vi "Get Error Counter Channels.vi"(8 "error in":errorcluster, 11 "status section in":T1 format="%.0x") -> (0 "error out":errorcluster, 2 "error counter channel refs":T2={"general protocol"=18446744073709551615, "improper number of words"=18446744073709551615, "Manchester"=18446744073709551615, "monitor"=18446744073709551615, "parity"=18446744073709551615, "unconfigured frames"=18446744073709551615, "word"=18446744073709551615, "wrong sync"=18446744073709551615} {"wrong sync" format="%.0x"; "word" format="%.0x"; "unconfigured frames" format="%.0x"; "parity" format="%.0x"; "monitor" format="%.0x"; "Manchester" format="%.0x"; "improper number of words" format="%.0x"; "general protocol" format="%.0x"}, 3 "status section out":T1 format="%.0x")   [LabVIEW 2020, in "Ballard MIL-STD-1553 Scripting.lvlib"]
uses:
  <vilib>/NI VeriStand/Custom Device API/Custom Device Item Ref.ctl
  Constants.vi
  Ballard MIL-STD-1553 Scripting.lvlib
  <vilib>/NI VeriStand/Custom Device Tools/Custom Device Utility Library/Custom Device Utility Library.lvlib
  <vilib>/NI VeriStand/Custom Device Tools/Custom Device Utility Library/NI VeriStand - Search for Item by Name.vi
  <vilib>/NI VeriStand/Custom Device API/Custom Device API.lvlib
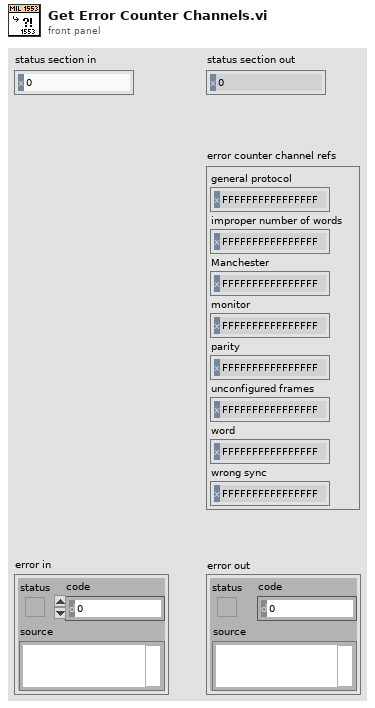
[diagram p1: front panel]
types:
  T1 = typedef "Custom Device API.lvlib/Custom Device Item Ref.ctl" = u64
  T2 = cluster{"general protocol":T1, "improper number of words":T1, "Manchester":T1, "monitor":T1, "parity":T1, "unconfigured frames":T1, "word":T1, "wrong sync":T1}
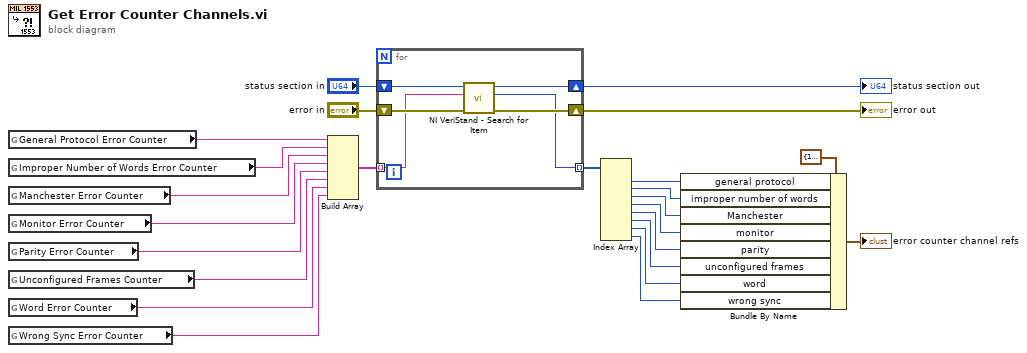
[diagram p0: block diagram]
diagram:
  n1 = global read "Constants.vi" "General Protocol Error Counter"() -> (w18:string)
  n2 = global read "Constants.vi" "Improper Number of Words Error Counter"() -> (w17:string)
  n3 = global read "Constants.vi" "Manchester Error Counter"() -> (w16:string)
  n4 = global read "Constants.vi" "Monitor Error Counter"() -> (w15:string)
  n5 = global read "Constants.vi" "Parity Error Counter"() -> (w14:string)
  n6 = global read "Constants.vi" "Unconfigured Frames Counter"() -> (w13:string)
  n7 = global read "Constants.vi" "Word Error Counter"() -> (w12:string)
  n8 = global read "Constants.vi" "Wrong Sync Error Counter"() -> (w11:string)
  n9 = Build Array(w18, w17, w16, w15, w14, w13, w12, w11) -> (w24:string[])
  n10 = for {
    shift-right: [w27] -> w20
    shift-left: "status section in" -> [w30]
    shift-right: [w28] -> w19
    shift-left: "error in" -> [w29]
    tunnel: w24 -> [w26] mode=indexing
    tunnel: [w25] -> w23 mode=indexing
    n11 = call-poly <vilib>:"NI VeriStand - Search for Item.vi"("error in"=w29, "Item Name"=w26, "Section Ref in"=w30) -> ("error out"=w28:errorcluster, "Item Ref"=w25:T1, "Section Ref out"=w27:T1)  [unwired: 5 in, 1 out]
  }
  "error out" <- w19
  "status section out" <- w20
  n12 = Index Array(array=w23) -> (element #1=w9:T1, element #2=w8:T1, element #3=w7:T1, element #4=w6:T1, element #5=w5:T1, element #6=w4:T1, element #7=w3:T1, element #8=w2:T1)  [unwired: 8 in]
  n13 = Bundle By Name(cluster=T2 {"general protocol"=18446744073709551615, "improper number of words"=18446744073709551615, "Manchester"=18446744073709551615, "monitor"=18446744073709551615, "parity"=18446744073709551615, "unconfigured frames"=18446744073709551615, "word"=18446744073709551615, "wrong sync"=18446744073709551615} ("error counter channel refs"), "general protocol"=w9, "improper number of words"=w8, "Manchester"=w7, "monitor"=w6, "parity"=w5, "unconfigured frames"=w4, "word"=w3, "wrong sync"=w2) -> (→"error counter channel refs":T2)
